vi "Controls and Q.vi"() -> ()   [LabVIEW 2021]
panel:
  in  "Numeric Control":i32
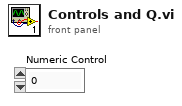
[diagram p1: front panel]
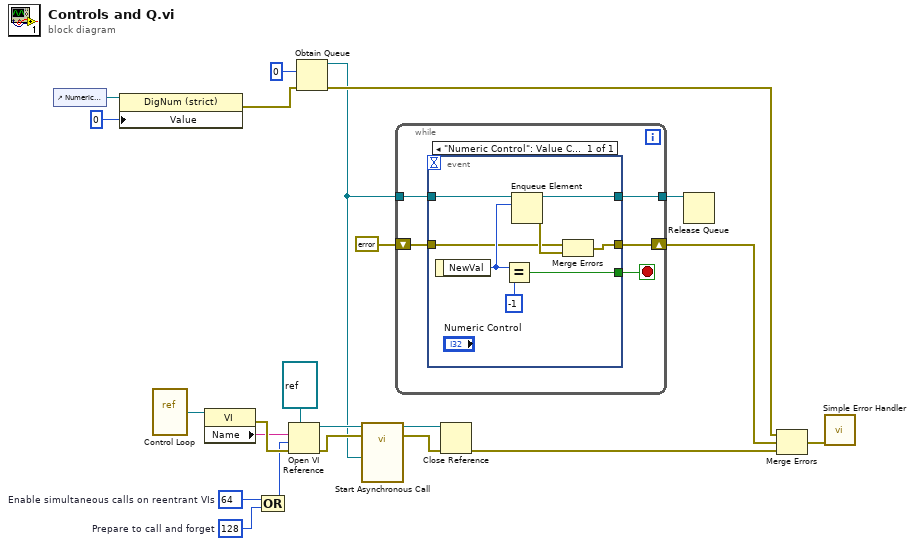
[diagram p0: block diagram]
diagram:
  w13 = 128  # Prepare to call and forget
  w14 = 64  # Enable simultaneous calls on reentrant VIs
  n1 = control-ref of="Numeric Control"() -> (w22:refnum<vi>)
  n2 = property class="DigNum (strict)"(reference=w22, "Value"=0) -> (error out=w5:errorcluster)  [unwired: 1 in, 1 out]
  n3 = vi-ref "Control Loop.vi"() -> (w17:refnum<vi>)
  n4 = property class="VI"(reference=w17) -> (error out=w16:errorcluster, "Name"=w15:string)  [unwired: 1 in, 1 out]
  n5 = Compound Arithmetic op=OR(w14, w13) -> (w12:i32)
  n6 = Open VI Reference(type specifier VI Refnum (for type only)=refnum<vi> refnum, vi path=w15, options=w12, error in (no error)=w16) -> (vi reference=w10:refnum<vi>, error out=w11:errorcluster)  [unwired: 2 in]
  n7 = Obtain Queue(element data type=0 ("I32"), error in (no error)=w5) -> (queue out=w2:refnum<queue>, error out=w9:errorcluster)  [unwired: 3 in, 1 out]
  n8 = call-by-ref "Start Asynchronous Call"(reference=w10, error in=w11, "Queue"=w2) -> (reference out=w6:refnum<vi>, error out=w8:errorcluster)  [unwired: 11 in]
  n9 = while {
    shift-right: [w26] -> w3
    shift-left: errorcluster {"status"=FALSE, "code"=0, "source"=""} ("error IO") -> [w25]
    tunnel: w2 -> [w24]
    tunnel: [w23] -> w1
    stop <- w27 stop-if-true
    n10 = event shown="[0] \"Numeric Control\": Value Change" {
      selector: _ -> [_]
      dyn-events: _ -> [_]
      timeout: _ -> [_]
      tunnel: w24 -> [w32]
      tunnel: [w34] -> w27
      tunnel: [w30] -> w26
      tunnel: w25 -> [w29]
      tunnel: [w28] -> w23
      event "Numeric Control": Value Change {
        n11 = event-data() -> ("NewVal"=w33:i32)  [unwired: 1 in]
        n12 = Equal?(x=w33, y=-1) -> (x = y?=w34:bool)
        n13 = Enqueue Element(queue=w32, element=w33) -> (queue out=w28:refnum<queue>, error out=w31:errorcluster)  [unwired: 2 in, 1 out]
        n14 = Merge Errors(w29, w31) -> (w30:errorcluster)
      }
    }
  }
  n15 = Close Reference(reference=w6, error in (no error)=w8) -> (error out=w7:errorcluster)
  n16 = Release Queue(queue=w1) -> ()  [unwired: 2 in, 3 out]
  n17 = Merge Errors(w9, w3, w7) -> (w19:errorcluster)
  n18 = call <vilib>:"Simple Error Handler.vi"("error in (no error)"=w19) -> ()  [unwired: 4 in, 5 out]
